vi "FPGA VI_Simulated_PeakandHold_Example.vi"() -> ()   [LabVIEW 2015]
uses:
  Types/Injection.Timing.ctl
  Types/Injection.Core.Settings.ctl
  Types/Injection.Global.Settings.ctl
  Types/Injection.Mux.State.ctl
  <vilib>/Platform/TimedLoop/XDataNode/timing_clust.ctl
  <vilib>/Platform/TimedLoop/XDataNode/nitl_modes.ctl
  <vilib>/Platform/TimedLoop/XDataNode/wakeup.ctl
  Types/Injection.Core.Internal.Settings.ctl
  <vilib>/rvi/DataTransferAndStorage/Container/Common/niFpgaContainerGetUniqueNameForEmu.vi
  <vilib>/rvi/DataTransferAndStorage/Container/Common/niFpgaContainerSetEmuInfo.vi
  <vilib>/rvi/eio/common/nirviEmuReportErrorAndStop.vi
  <vilib>/rvi/Emulation/niFpgaGetClockAttributes.vi
  <vilib>/rvi/Emulation/niFpgaSctlEmulationGetInTimedLoop.vi
  <vilib>/rvi/Emulation/niFpgaEmulationReportErrorSimple.vi
  <vilib>/rvi/Memory/Memory_Emulation/nirvimemoryFastEmulation.vi
  <vilib>/rvi/Memory/Memory_Emulation/nirvimemoryEmulation.vi
  <vilib>/rvi/Emulation/niFpgaEmulationIsFPGAContextNoSignature.vi
  <vilib>/rvi/Emulation/niFpgaProcessEmulError.vi
  <vilib>/rvi/errors/nirviReportUnexpectedCaseInternalError (U32).vi
  <vilib>/rvi/Emulation/niFpgaCriticalErrorInLSC.vi
  <vilib>/rvi/DataTransferAndStorage/Container/Common/niFpgaContainerExecOnDevCompGetState.vi
  <vilib>/rvi/errors/niFpgaSetErrorForExecOnDevCompSimple.vi
  <vilib>/rvi/FIFO/Fifo_Resource/nirvififoEmulationSetSize.vi
  <vilib>/rvi/FIFO/Fifo_Resource/nirviFifoEmulationQueueMgr.vi
  <instcachedir>/0/nirviFifoEmulationQueueMgr_E5CAEC123FF24DC58D834DCA3CDAA9B5.lvgen/nirviFifoEmulationQueueMgr_E5CAEC123FF24DC58D834DCA3CDAA9B5_010.vi
  <vilib>/rvi/FIFO/Fifo_Resource/nirvififoEmulationDetermineInputValidOut.vi
  <vilib>/rvi/FIFO/Fifo_Resource/nirvififoEmulationCreateLock.vi
  <vilib>/rvi/FIFO/Fifo_Resource/nirvififoEmulationObtainLock.vi
  <vilib>/rvi/FIFO/Fifo_Resource/nirvififoEmulationReleaseLock.vi
  <vilib>/rvi/occurrence/nirviWaitOnOccurrenceBase.vi
  <vilib>/rvi/errors/nirviReportUnexpectedCaseInternalError.vi
  <vilib>/Utility/error.llb/Clear Errors.vi
  <vilib>/rvi/interface/RandomDataEmulation/niFpgaRandomDataHandleErrors.vi
  <instcachedir>/0/nirviFifoEmulationQueueMgr_E5CAEC123FF24DC58D834DCA3CDAA9B5.lvgen/nirviFifoEmulationQueueMgr_E5CAEC123FF24DC58D834DCA3CDAA9B5_008.vi
  <vilib>/rvi/LocalResourceManager/LocalResourceManager.xnode
  <vilib>/rvi/DataTransferAndStorage/Container/XNode/niFpgaContainer.xnode
  <vilib>/Platform/TimedLoop/XDataNode/XDataNode.xnode
  <vilib>/rvi/FIFO/Fifo_Resource/niFpgaFifoEmulationRefIn.vi
  <vilib>/rvi/interface/RandomDataEmulation/nirviRandomDataFpgaReadWriteTemplate.vi
  <vilib>/Platform/TimedLoop/XDataNode/XDNodeRunTimeDep.lvlib
panel:
  in  "Settings.Global.PeakAndHoldHS":T1={"Enable?"=FALSE, "Initial Voltage Threshold"=12.0, "Event Dwell Limit"=2000, "Voltage Gain"=1.0, "Current Gain"=1.0, "Filter Samples"=5, "Pretrigger Samples"=5}
  in  "Settings.Index1.PeakAndHoldHS.HS":T2
  out "Intermediate FIFO Write Timeout":bool
  in  "Settings.Global.PeakAndHoldLS":T1={"Enable?"=FALSE, "Initial Voltage Threshold"=12.0, "Event Dwell Limit"=2000, "Voltage Gain"=1.0, "Current Gain"=1.0, "Filter Samples"=5, "Pretrigger Samples"=5}
  in  "Settings.Index0.PeakAndHoldLS.LS":T2
  in  "Settings.Timing":T3={"Injection Sample Period (Ticks)"=80}
  out "Acqusition Loop Ticks":u32
  in  "Settings.DMA":cluster{"# of Injectors":u8}={"# of Injectors"=2}
  out "Host DMA Out?":bool
  out "Intermediate Time Out?":bool
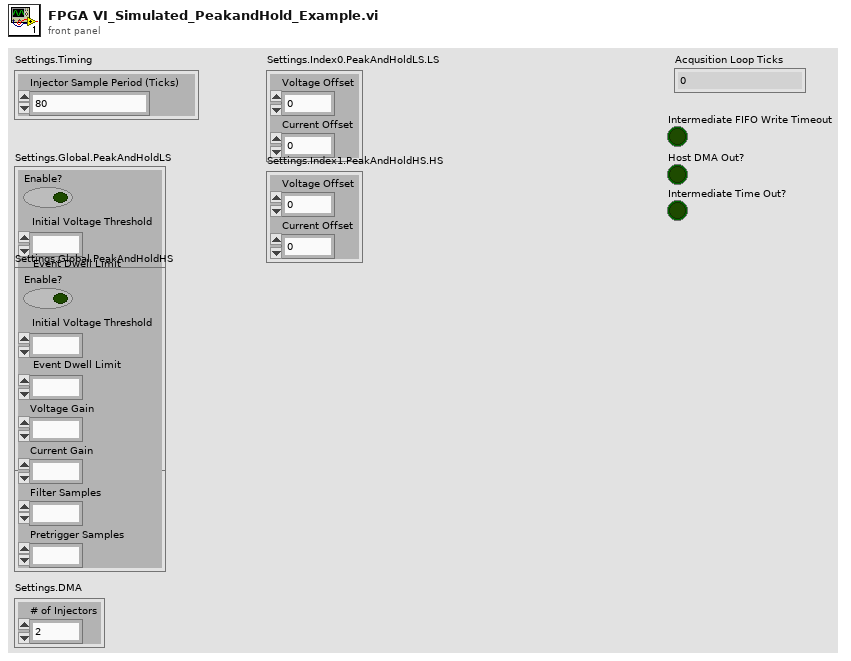
[diagram p1: front panel]
types:
  T1 = typedef "Injection.Global.Settings.ctl" = cluster{"Enable?":bool, "Initial Voltage Threshold":fxp<+/-,32,8>, "Event Dwell Limit":u16, "Voltage Gain":fxp<+/-,32,8>, "Current Gain":fxp<+/-,32,8>, "Filter Samples":u8, "Pretrigger Samples":u8}
  T2 = typedef "Injection.Core.Settings.ctl" = cluster{"Voltage Offset":fxp<+/-,32,8>, "Current Offset":fxp<+/-,32,8>}
  T3 = typedef "Injection.Timing.ctl" = cluster{"Injection Sample Period (Ticks)":u32}
  T4 = cluster{"Data.Samples":u32, "Injection.Period":u32, "Injector.Index":u8, "Iteration":u32}
  T5 = typedef "Injection.Mux.State.ctl" = enum8{"Wait on Transfer", "Transfer Injector Index", "Transfer # of Samples", "Transfer Injection Period", "Transfer Data Samples"}
  T6 = typedef "XDNodeRunTimeDep.lvlib/timing_clust.ctl" = cluster{"Expected End [f-1]":u64, "Actual End [f-1]":u64, "Finished Late? [f-1]":bool, "Expected End [i-1]":u64, "Actual End [i-1]":u64, "Finished Late? [i-1]":bool, "Expected Start [i]":u64, "Actual Start [i]":u64, "Expected Start [f]":u64, "Actual Start [f]":u64, "Source Name":string, "Structure Name":string, "Period":i64, "Deadline":i64, "Offset":i64, "Start":i64, "Priority":i32, "Timeout":i32, "Mode":T7, "Wakeup Reason":T8, "Error":errorcluster, "Source Type":string, "Secondary Source Type":string, "Global End Time":u64, "Global Start Time":u64, "Frame Duration":u64, "Iteration Duration":u64, "Assigned CPU":i32, "I/O Scan Engine Mode":u32}
  T7 = typedef "XDNodeRunTimeDep.lvlib/nitl_modes.ctl" = enum32{"No Change", "Process missed periods, maintain original phase", "Discard missed periods, maintain original phase", "Process missed periods, ignore original phase", "Discard missed periods, ignore original phase"}
  T8 = typedef "XDNodeRunTimeDep.lvlib/wakeup.ctl" = enum32{"Normal", "Aborted", "Asynchronous wakeup", "Timing source error", "Timed loop error", "Timeout"}
  T9 = typedef "Injection.Core.Internal.Settings.ctl" = cluster{"Data Buffer FIFO":refnum<k21>, "Capture Complete Trigger FIFO":refnum<k21>}
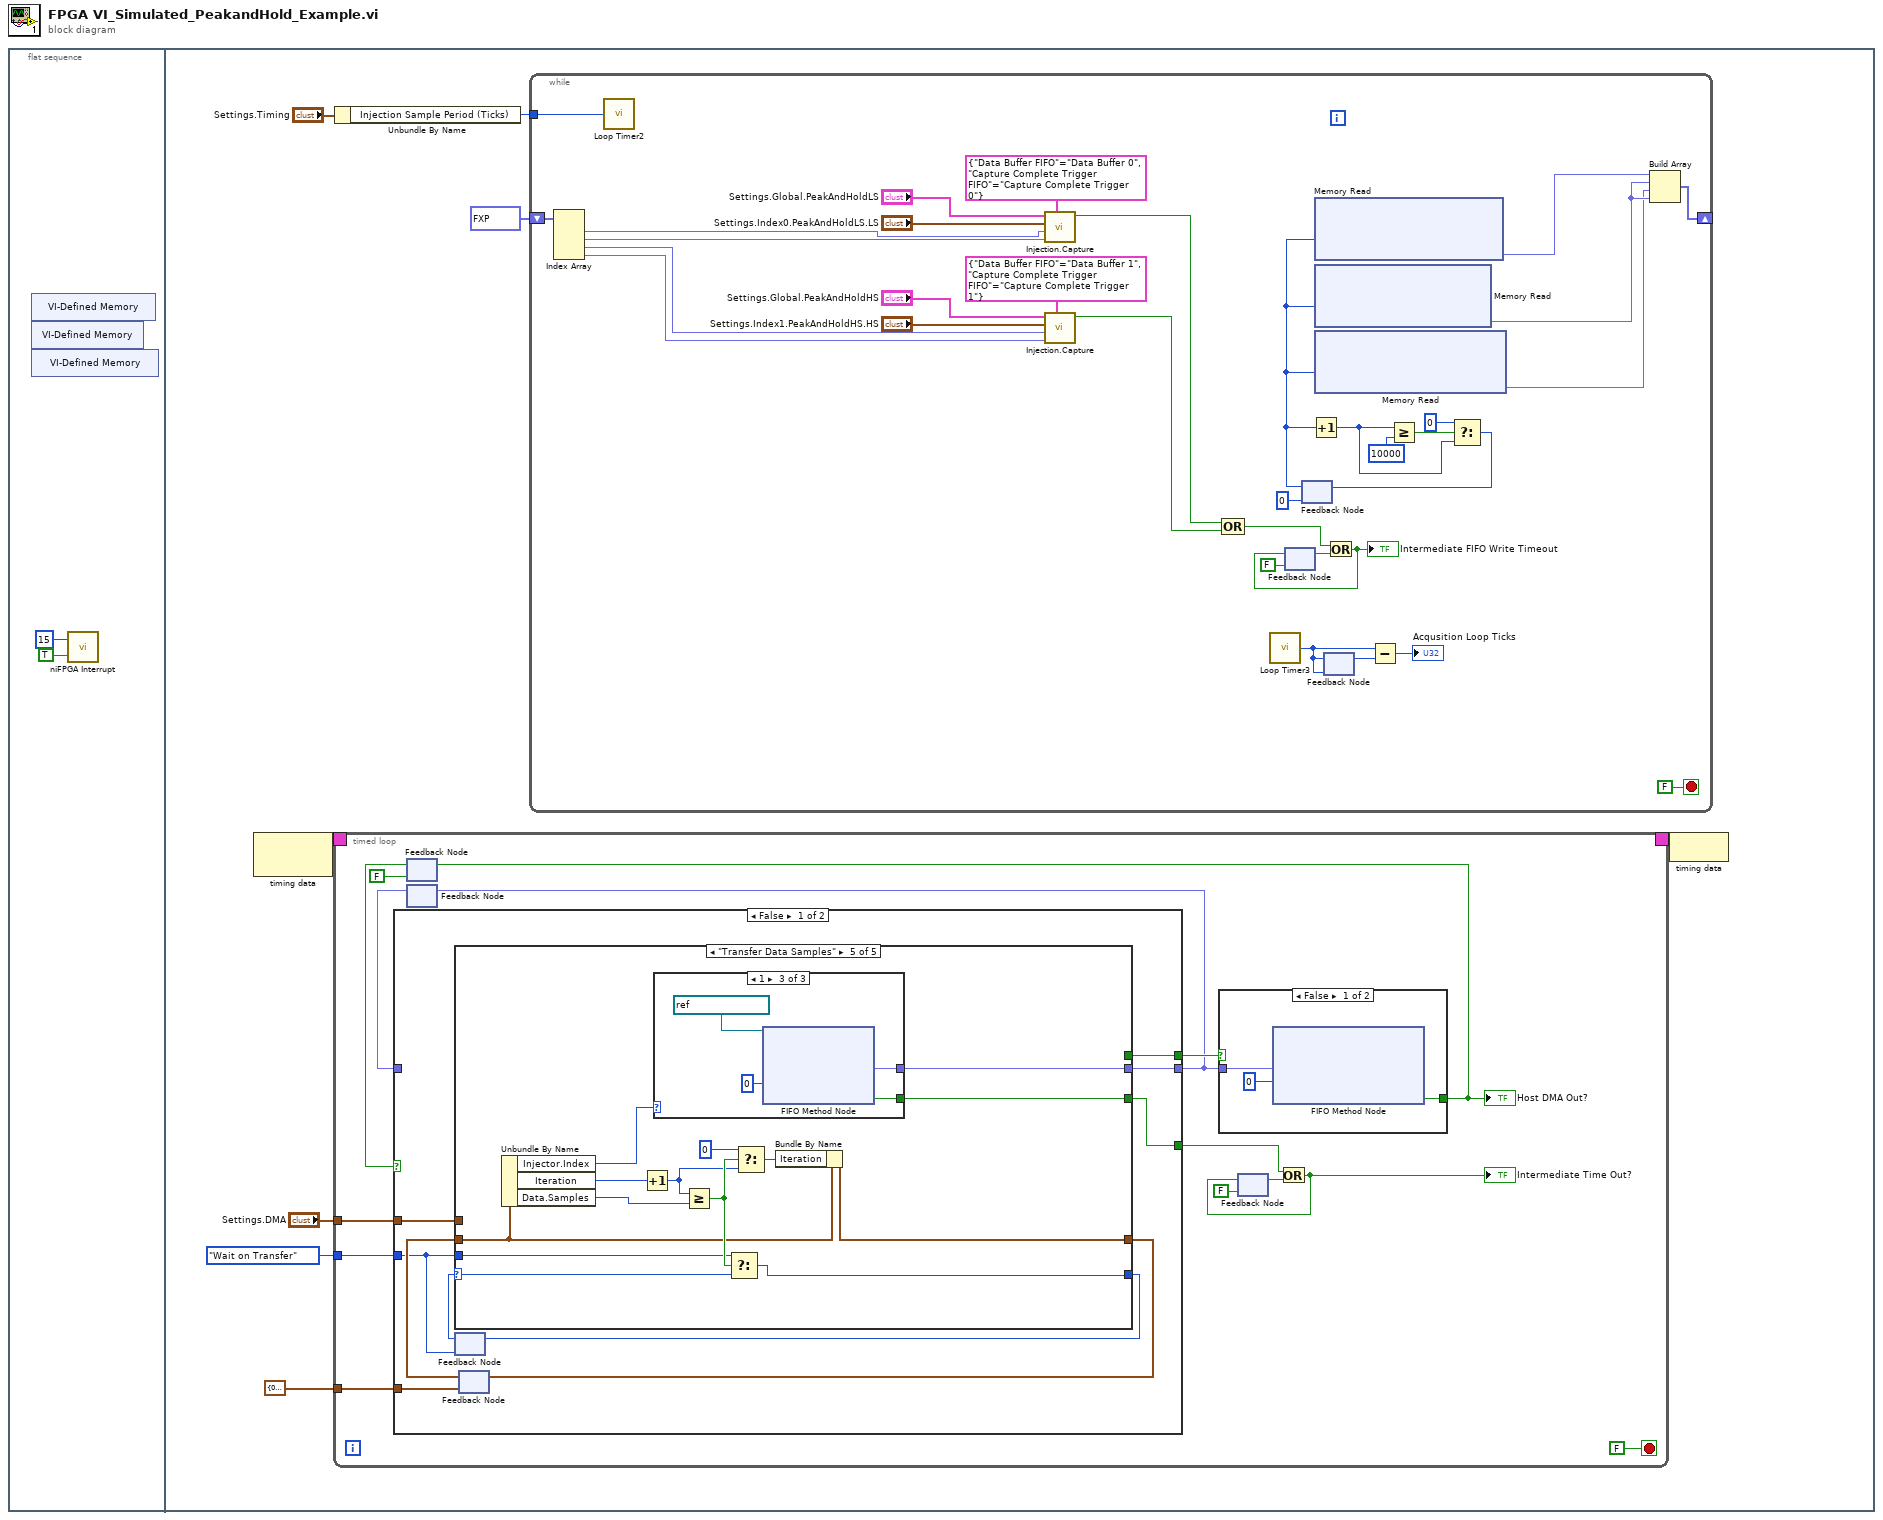
[diagram p0: block diagram]
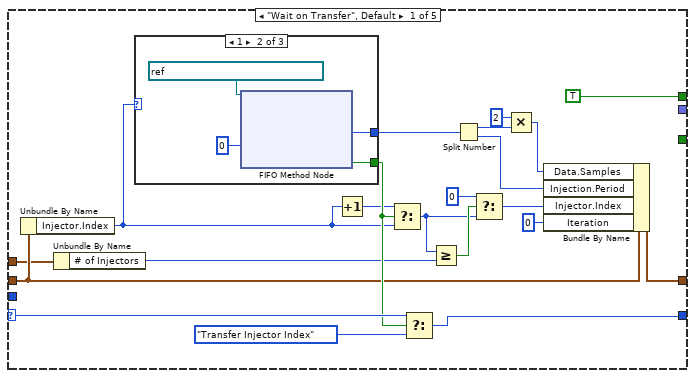
[diagram p2: hidden frame]
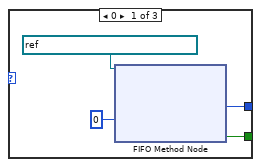
[diagram p3: hidden frame]
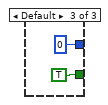
[diagram p4: hidden frame]
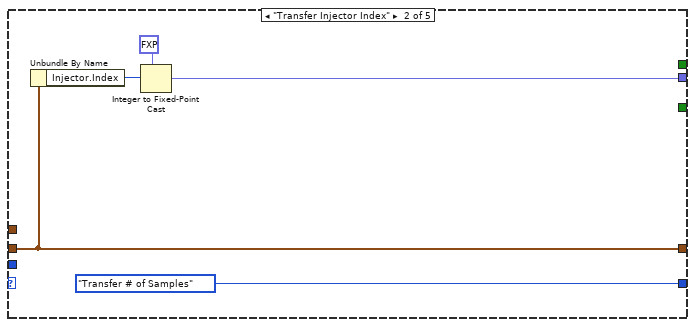
[diagram p5: hidden frame]
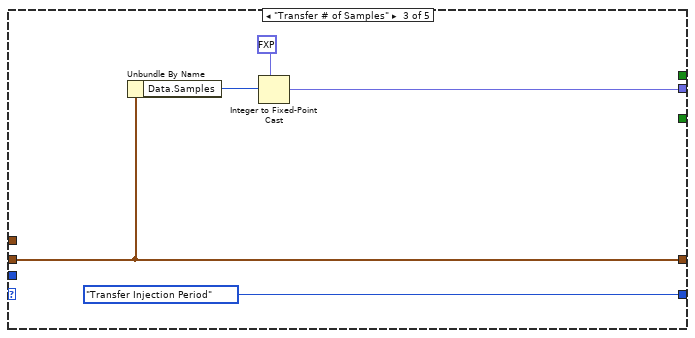
[diagram p6: hidden frame]
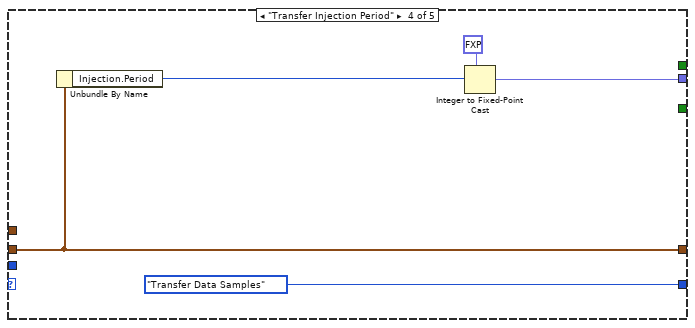
[diagram p7: hidden frame]
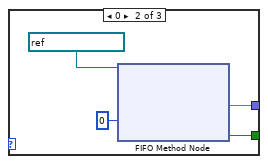
[diagram p9: hidden frame]
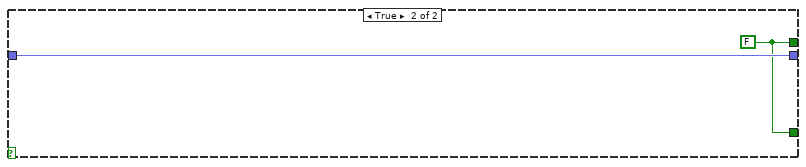
[diagram p10: hidden frame]
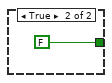
[diagram p11: hidden frame]
diagram:
  n1 = flat-sequence {
    frame #0 {
      n2 = xnode "VI-Defined Memory"() -> ()  [unwired: 1 out]
      n3 = xnode "VI-Defined Memory"() -> ()  [unwired: 1 out]
      n4 = xnode "VI-Defined Memory"() -> ()  [unwired: 1 out]
      n5 = call <vilib>:"niFPGA Interrupt.vi"("Wait Until Cleared (F)"=TRUE, "IRQ Number (0)"=u8 15) -> ()  [unwired: 1 in]
    }
    frame #1 {
      n6 = node-c288() -> (w10:T6)  [unwired: 1 in]
      n7 = timed-loop {
        timing: w10 -> [_]
        timing-out: [_] -> w9
        tunnel: "Settings.DMA" -> [w14]
        tunnel: Injection.Mux.State."Wait on Transfer" -> [w13]
        tunnel: T4 {"Data.Samples"=0, "Injection.Period"=0, "Injector.Index"=0, "Iteration"=0} ("Local.Data") -> [w12]
        stop <- FALSE stop-if-true
        n8 = feedback #1(FALSE ("Timed Out?")) -> (w22:bool)
        n9 = feedback #2() -> (w19:fxp<+/-,32,8>)  [unwired: 1 in]
        n10 = case shown="False" w22 {
          tunnel: [w34 w104] -> w20
          tunnel: [w33 w103] -> w24
          tunnel: w13 -> [w27 _]
          tunnel: [w32 w103] -> w15
          tunnel: w14 -> [w31 _]
          tunnel: w12 -> [w28 _]
          tunnel: w19 -> [_ w104]
          frame False {
            n11 = feedback #3(w27) -> (w26:T5)
            n12 = feedback #4(w28) -> (w29:T4)
            n13 = case shown="\"Transfer Data Samples\"" w26 {
              selector: w26 -> [w55 _ _ _ w88]
              tunnel: w29 -> [w46 w69 w73 w77 w86]
              tunnel: [w54 w69 w73 w77 w85] -> w30
              tunnel: [w53 Injection.Mux.State."Transfer # of Samples" Injection.Mux.State."Transfer Injection Period" Injection.Mux.State."Transfer Data Samples" w87] -> w25
              tunnel: [_ w68 w72 w79 w84] -> w34
              tunnel: [TRUE _ _ _ _] -> w33
              tunnel: w27 -> [_ _ _ _ w81]
              tunnel: [_ _ _ _ w83] -> w32
              tunnel: w31 -> [w43 _ _ _ _]
              frame "Wait on Transfer", Default {
                n14 = Unbundle By Name(w46) -> ("Injector.Index"=w45:u8)
                n15 = Unbundle By Name(w43) -> ("# of Injectors"=w42:u8)
                n16 = case shown="1" w45 {
                  tunnel: [w58 w62 u64 0 ("Element")] -> w41
                  tunnel: [w57 w61 TRUE ("Timed Out?")] -> w51
                  frame 0 {
                    n17 = xnode ("FIFO Method Node")("Timeout"=0, "FIFO In"=refnum<k21> "Capture Complete Trigger 0") -> ("Element"=w58:u64, "Timed Out?"=w57:bool)  [unwired: 1 out]
                  }
                  frame 1 {
                    n18 = xnode ("FIFO Method Node")("Timeout"=0, "FIFO In"=refnum<k21> "Capture Complete Trigger 1") -> ("Element"=w62:u64, "Timed Out?"=w61:bool)  [unwired: 1 out]
                  }
                  frame Default {
                  }
                }
                n19 = Increment(x=w45) -> (x+1=w50:u8)
                n20 = Select(t=w50, s=w51, f=w45) -> (s? t:f=w48:u8)
                n21 = Select(t=w55, s=w51, f=Injection.Mux.State."Transfer Injector Index") -> (s? t:f=w53:T5)
                n22 = Greater Or Equal?(x=w48, y=w42) -> (x >= y?=w49:bool)
                n23 = Split Number(x=w41) -> (hi(x)=w40:u32, lo(x)=w39:u32)
                n24 = Select(t=u8 0, s=w49, f=w48) -> (s? t:f=w44:u8)
                n25 = Multiply(x=u32 2, y=w40) -> (x*y=w37:u32)
                n26 = Bundle By Name(cluster=w46, "Data.Samples"=w37, "Injection.Period"=w39, "Injector.Index"=w44, "Iteration"=u32 0) -> (w54:T4)
              }
              frame "Transfer Injector Index" {
                n27 = Unbundle By Name(w69) -> ("Injector.Index"=w70:u8)
                n28 = Integer to Fixed-Point Cast(fixed-point type=fxp<+/-,32,8> 0.0, integer=w70) -> (fixed-point=w68:fxp<+/-,32,8>)
              }
              frame "Transfer # of Samples" {
                n29 = Unbundle By Name(w73) -> ("Data.Samples"=w74:u32)
                n30 = Integer to Fixed-Point Cast(fixed-point type=fxp<+/-,32,8> 0.0, integer=w74) -> (fixed-point=w72:fxp<+/-,32,8>)
              }
              frame "Transfer Injection Period" {
                n31 = Unbundle By Name(w77) -> ("Injection.Period"=w78:u32)
                n32 = Integer to Fixed-Point Cast(fixed-point type=fxp<+/-,32,8> 0.0, integer=w78) -> (fixed-point=w79:fxp<+/-,32,8>)
              }
              frame "Transfer Data Samples" {
                n33 = Unbundle By Name(w86) -> ("Injector.Index"=w94:u8, "Iteration"=w89:u32, "Data.Samples"=w82:u32)
                n34 = Increment(x=w89) -> (x+1=w91:u32)
                n35 = case shown="1" w94 {
                  tunnel: [_ w97 w101] -> w84
                  tunnel: [_ w96 w100] -> w83
                  frame Default {
                  }
                  frame 0 {
                    n36 = xnode ("FIFO Method Node")("Timeout"=0, "FIFO In"=refnum<k21> "Data Buffer 0" ("Voltage FIFO")) -> ("Element"=w97:fxp<+/-,32,8>, "Timed Out?"=w96:bool)  [unwired: 1 out]
                  }
                  frame 1 {
                    n37 = xnode ("FIFO Method Node")("Timeout"=0, "FIFO In"=refnum<k21> "Data Buffer 1" ("Voltage FIFO")) -> ("Element"=w101:fxp<+/-,32,8>, "Timed Out?"=w100:bool)  [unwired: 1 out]
                  }
                }
                n38 = Greater Or Equal?(x=w91, y=w82) -> (x >= y?=w93:bool)
                n39 = Select(t=w81, s=w93, f=w88) -> (s? t:f=w87:T5)
                n40 = Select(t=u32 0, s=w93, f=w91) -> (s? t:f=w90:u32)
                n41 = Bundle By Name(cluster=w86, "Iteration"=w90) -> (w85:T4)
              }
            }
            n42 = feedback-in #3(w25) -> ()
            n43 = feedback-in #4(w30) -> ()
          }
          frame True {
            w103 = FALSE
          }
        }
        n44 = feedback-in #2(w20) -> ()
        n45 = case shown="False" w24 {
          tunnel: w20 -> [w106 _]
          tunnel: [w105 FALSE ("Timed Out?")] -> w23
          frame False {
            n46 = xnode ("FIFO Method Node")("Element"=w106, "Timeout"=0) -> ("Timed Out?"=w105:bool)  [unwired: 1 in, 1 out]
          }
          frame True {
          }
        }
        "Host DMA Out?" <- w23
        n47 = feedback-in #1(w23) -> ()
        n48 = feedback #5(FALSE ("Timed Out?")) -> (w17:bool)
        n49 = Or(x=w15, y=w17) -> (x .or. y?=w16:bool)
        "Intermediate Time Out?" <- w16
        n50 = feedback-in #5(w16) -> ()
      }
      n51 = Unbundle By Name("Settings.Timing") -> ("Injection Sample Period (Ticks)"=w3:u32)
      n52 = while {
        shift-right: [w124] -> _
        shift-left: fxp<+/-,32,8>[] [0.0, 0.0, 0.0, 0.0] -> [w142]
        tunnel: w3 -> [w131]
        stop <- FALSE stop-if-true
        n53 = Index Array(array=w142) -> (element #1=w122:fxp<+/-,32,8>, element #2=w143:fxp<+/-,32,8>, element #3=w118:fxp<+/-,32,8>, element #4=w117:fxp<+/-,32,8>)  [unwired: 4 in]
        n54 = call "Loop Timer2"("Count(Ticks)"=w131) -> ()  [unwired: 1 out]
        n55 = call "Injection.Capture.vi"("FIFOs"=T9 {"Data Buffer FIFO"="Data Buffer 0", "Capture Complete Trigger FIFO"="Capture Complete Trigger 0"} ("InjectorCore.Settings"), "Current (PreScaled)"=w143, "Voltage (PreScaled)"=w122, "Settings.Index<#>.<Group>.<UserName>"="Settings.Index0.PeakAndHoldLS.LS", "Settings.Global.<Group>"="Settings.Global.PeakAndHoldLS") -> ("Intermediate FIFO Timeout?"=w145:bool)  [unwired: 4 in, 2 out]
        n56 = call "Injection.Capture.vi"("FIFOs"=T9 {"Data Buffer FIFO"="Data Buffer 1", "Capture Complete Trigger FIFO"="Capture Complete Trigger 1"} ("InjectorCore.Settings"), "Current (PreScaled)"=w117, "Voltage (PreScaled)"=w118, "Settings.Index<#>.<Group>.<UserName>"="Settings.Index1.PeakAndHoldHS.HS", "Settings.Global.<Group>"="Settings.Global.PeakAndHoldHS") -> ("Intermediate FIFO Timeout?"=w115:bool)  [unwired: 4 in, 2 out]
        n57 = Compound Arithmetic op=OR(w145, w115) -> (w136:bool)
        n58 = call "Loop Timer3"() -> ("Tick Count(Ticks)"=w132:u32)  [unwired: 1 in]
        n59 = feedback #6(FALSE ("Timed Out?")) -> (w137:bool)
        n60 = feedback #7(u32 0 ("Address")) -> (w114:u32)
        n61 = Increment(x=w114) -> (x+1=w127:u32)
        n62 = xnode ("Memory Read")("Address"=w114) -> ("Data"=w123:fxp<+/-,32,8>)  [unwired: 1 in, 1 out]
        n63 = xnode ("Memory Read")("Address"=w114) -> ("Data"=w116:fxp<+/-,32,8>)  [unwired: 1 in, 1 out]
        n64 = xnode ("Memory Read")("Address"=w114) -> ("Data"=w113:fxp<+/-,32,8>)  [unwired: 1 in, 1 out]
        n65 = feedback-in #8(w132) -> ()
        n66 = feedback #8(w132) -> (w134:u32)
        n67 = Or(x=w136, y=w137) -> (x .or. y?=w135:bool)
        "Intermediate FIFO Write Timeout" <- w135
        n68 = feedback-in #6(w135) -> ()
        n69 = Subtract(x=w132, y=w134) -> (x-y=→"Acqusition Loop Ticks":u32)
        n70 = Greater Or Equal?(x=w127, y=u32 10000) -> (x >= y?=w126:bool)
        n71 = Select(t=u32 0, s=w126, f=w127) -> (s? t:f=w129:u32)
        n72 = feedback-in #7(w129) -> ()
        n73 = Build Array(w123, w116, w113, w116) -> (w124:fxp<+/-,32,8>[])
      }
      n74 = node-c288(w9) -> ()
    }
  }
